vi "PH_SRDG645.get Channel.vi"(0 "i ref in":refnum<vi>, 1 "Channel (T0)":T1 items=["T0", "T1", "A", "B", "C", "D", "E", "F", "G", "H"], 5 "error IO":errorcluster) -> (14 "i ref out":refnum<vi>, 19 "error out":errorcluster)   [LabVIEW 2014, in "PH_SRDG645.lvlib"]
doc: "This VI querries the channel settings from the hardware."
uses:
  PH_SRDG645.lvlib
  PH_SRDG645.Channel Settings.ctl
  instr.lib/SRDG645/Driver/Channel.ctl
  instr.lib/SRDG645/Stanford Research DG645 - Driver.lvlib
panel:
  in  "Channel cluster":T2={"Delay [s]"=0.0, "relative to"=1000} {"relative to" items=["T0", "T1", "A", "B", "C", "D", "E", "F", "G", "H"]; "Delay [s]" format="%#_12p"}
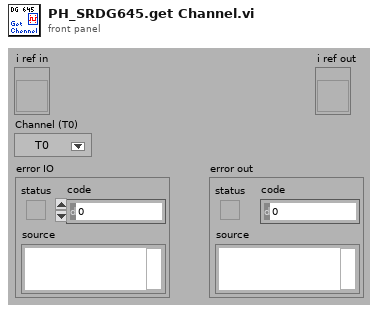
[diagram p1: front panel]
types:
  T1 = typedef "Stanford Research DG645 - Driver.lvlib/Channel.ctl" = i32
  T2 = typedef "PH_SRDG645.lvlib/PH_SRDG645.Channel Settings.ctl" = cluster{"Delay [s]":dbl, "relative to":i32}
  T3 = typedef "PH_SRDG645.lvlib/PH_SRDG645.i attribute.ctl" = cluster{"GUI Refs":cluster{"Delete":refnum<vi>, "Device Errors":refnum<vi>, "Trigger":refnum<vi>, "Default Name":refnum<vi>, "Firmware Revision":refnum<vi>, "Serial Number":refnum<vi>, "Model":refnum<vi>, "Visa resource name":refnum<vi>}, "Service ID Rate":i32, "Service IDs Channelinfo":i32[], "VISA resource name":refnum<visa-resource-name>, "Device Errors":cluster{"code":i32, "Text":string}[], "Trigger":T4, "Channels":cluster{"T1":T2, "A":T2, "B":T2, "C":T2, "D":T2, "E":T2, "F":T2, "G":T2, "H":T2}, "GUI Refs Channels":refnum<vi>[], "Outputs":cluster{"AB":cluster{"Level Offset [V]":dbl, "Amplitue [V]":dbl, "Polarity":i32}, "CD":cluster{"Level Offset [V]":dbl, "Amplitue [V]":dbl, "Polarity":i32}, "EF":cluster{"Level Offset [V]":dbl, "Amplitue [V]":dbl, "Polarity":i32}, "GH":cluster{"Level Offset [V]":dbl, "Amplitue [V]":dbl, "Polarity":i32}, "T0":cluster{"Level Offset [V]":dbl, "Amplitue [V]":dbl, "Polarity":i32}}, "GUI Refs Outputs":refnum<vi>[], "Serial Number":string, "Firmweare Revision":string, "Model":string}
  T4 = typedef "PH_SRDG645.lvlib/PH_SRDG645.Trigger.ctl" = cluster{"Source":i32, "Rate [Hz]":dbl, "Level [V]":dbl}
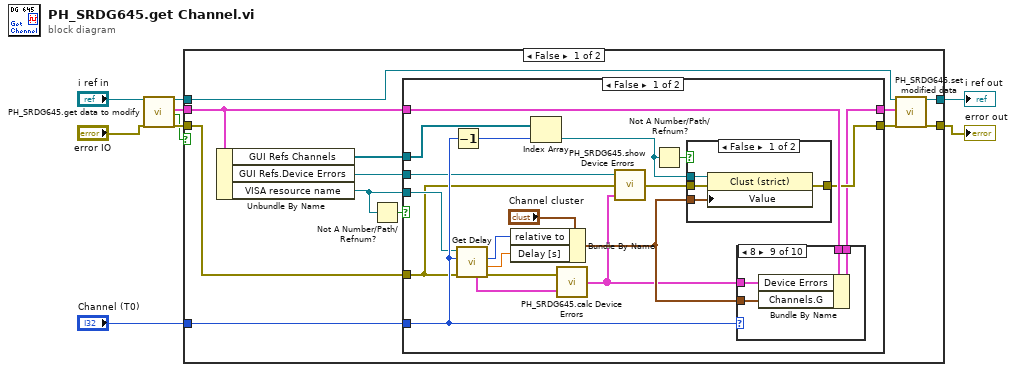
[diagram p0: block diagram]
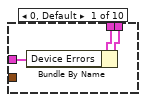
[diagram p2: hidden frame]
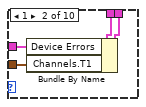
[diagram p3: hidden frame]
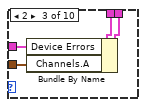
[diagram p4: hidden frame]
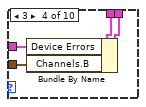
[diagram p5: hidden frame]
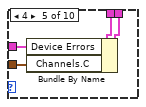
[diagram p6: hidden frame]
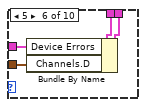
[diagram p7: hidden frame]
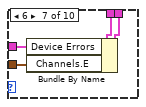
[diagram p8: hidden frame]
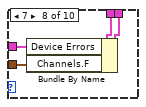
[diagram p9: hidden frame]
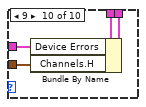
[diagram p10: hidden frame]
diagram:
  n1 = call "PH_SRDG645.get data to modify.vi"("i ref in"="i ref in", "error in (no error)"="error IO") -> ("i ref out"=w7:refnum<vi>, "i attribute"=w4:T3, "timed out"=w2:bool, "error out"=w5:errorcluster)  [unwired: 14 in]
  n2 = case shown="False" w2 {
    tunnel: w7 -> [w10 w88]
    tunnel: [w14 w88] -> w6
    tunnel: w5 -> [w18 w87]
    tunnel: w4 -> [w21 _]
    tunnel: [w12 w87] -> w3
    tunnel: "Channel (T0)" -> [w17 _]
    frame False {
      n3 = Unbundle By Name(w21) -> ("GUI Refs Channels"=w20:refnum<vi>[], "GUI Refs.Device Errors"=w19:refnum<vi>, "VISA resource name"=w16:refnum<visa-resource-name>)
      n4 = Not A Number/Path/Refnum?(number/path/refnum=w16) -> (NaN/Path/Refnum?=w15:bool)
      n5 = case shown="False" w15 {
        tunnel: w21 -> [w39 w85]
        tunnel: [w29 w86] -> w13
        tunnel: w20 -> [w37 _]
        tunnel: w19 -> [w25 _]
        tunnel: w18 -> [w22 w86]
        tunnel: w17 -> [w31 _]
        tunnel: w16 -> [w30 _]
        tunnel: [w28 w85] -> w11
        frame False {
          n6 = Decrement(x=w31) -> (x-1=w35:T1)
          n7 = call "Get Delay.vi"("error in (no error)"=w22, "Channel (T0)"=w31, "VISA resource name"=w30) -> ("error out"=w23:errorcluster, "Delay [s]"=w33:dbl, "relative to"=w32:T1, "Device Errors"=w27:cluster{"code":i32, "Text":string}[])  [unwired: 4 in, 1 out]
          n8 = Bundle By Name(cluster="Channel cluster", "relative to"=w32, "Delay [s]"=w33) -> (w34:T2)
          n9 = Index Array(array=w37, index=w35) -> (element=w36:refnum<vi>)
          n10 = call "PH_SRDG645.calc Device Errors.vi"("Device Errors out"=w27, "SRDG 645 error out"=w23) -> ("calculate Device Errors"=w26:cluster{"code":i32, "Text":string}[])
          n11 = call "PH_SRDG645.show Device Errors.vi"("Device Errors"=w26, "error in"=w22, "Ref Device Errors"=w25) -> ("error out"=w24:errorcluster)
          n12 = Not A Number/Path/Refnum?(number/path/refnum=w36) -> (NaN/Path/Refnum?=w38:bool)
          n13 = case shown="False" w38 {
            tunnel: w36 -> [w83 _]
            tunnel: w34 -> [w82 _]
            tunnel: w24 -> [w81 w84]
            tunnel: [w80 w84] -> w29
            frame False {
              n14 = property class="Clust (strict)"(reference=w83, error in=w81, "Value"=w82) -> (error out=w80:errorcluster)  [unwired: 1 out]
            }
            frame True {
            }
          }
          n15 = case shown="8" w31 {
            tunnel: w39 -> [w43 w47 w51 w55 w59 w63 w67 w71 w75 w79]
            tunnel: [w41 w46 w50 w54 w58 w62 w66 w70 w74 w78] -> w28
            tunnel: w34 -> [_ w45 w49 w53 w57 w61 w65 w69 w73 w77]
            tunnel: w26 -> [w42 w44 w48 w52 w56 w60 w64 w68 w72 w76]
            frame 0, Default {
              n16 = Bundle By Name(cluster=w43, "Device Errors"=w42) -> (w41:T3)
            }
            frame 1 {
              n17 = Bundle By Name(cluster=w47, "Device Errors"=w44, "Channels.T1"=w45) -> (w46:T3)
            }
            frame 2 {
              n18 = Bundle By Name(cluster=w51, "Device Errors"=w48, "Channels.A"=w49) -> (w50:T3)
            }
            frame 3 {
              n19 = Bundle By Name(cluster=w55, "Device Errors"=w52, "Channels.B"=w53) -> (w54:T3)
            }
            frame 4 {
              n20 = Bundle By Name(cluster=w59, "Device Errors"=w56, "Channels.C"=w57) -> (w58:T3)
            }
            frame 5 {
              n21 = Bundle By Name(cluster=w63, "Device Errors"=w60, "Channels.D"=w61) -> (w62:T3)
            }
            frame 6 {
              n22 = Bundle By Name(cluster=w67, "Device Errors"=w64, "Channels.E"=w65) -> (w66:T3)
            }
            frame 7 {
              n23 = Bundle By Name(cluster=w71, "Device Errors"=w68, "Channels.F"=w69) -> (w70:T3)
            }
            frame 8 {
              n24 = Bundle By Name(cluster=w75, "Device Errors"=w72, "Channels.G"=w73) -> (w74:T3)
            }
            frame 9 {
              n25 = Bundle By Name(cluster=w79, "Device Errors"=w76, "Channels.H"=w77) -> (w78:T3)
            }
          }
        }
        frame True {
        }
      }
      n26 = call "PH_SRDG645.set modified data.vi"("i ref in"=w10, "i attribute"=w11, "error in (no error)"=w13) -> ("i ref out"=w14:refnum<vi>, "error out"=w12:errorcluster)  [unwired: 15 in]
    }
    frame True {
    }
  }
  "error out" <- w3
  "i ref out" <- w6
